vi "Mutate Multi FPGA.vi"(6 "Force (F)":bool, 8 "error in (no error)":errorcluster, 11 "Device Ref in":T1 format="%.0x") -> (0 "error out":errorcluster, 3 "Device Ref out":T1 format="%.0x")   [LabVIEW 2015, in "Engine Simulation Toolkit System Explorer.lvlib"]
uses:
  Engine Simulation Toolkit System Explorer.lvlib
  <vilib>/NI Veristand/Custom Device API/Custom Device Item Ref.ctl
  Shared/Channel.ctl
  <vilib>/NI Veristand/Custom Device API/Custom Device Channel Type.ctl
  Shared/Properties.vi
  Shared/Constants and GUIDs.vi
  <vilib>/NI Veristand/Custom Device API/Get Item Property (Boolean).vi
  <vilib>/NI Veristand/Custom Device API/Get Item Property (String).vi
  <vilib>/NI Veristand/Custom Device API/Set Item Property (String Array).vi
  <vilib>/NI Veristand/Custom Device API/Get Item Property (Dependent File).vi
  <vilib>/NI Veristand/Custom Device API/Set Item Property (String).vi
  <vilib>/NI Veristand/Custom Device Tools/Custom Device Utility Library/NI VeriStand - Search for All Items by GUID.vi
  <vilib>/NI Veristand/Custom Device API/Set Item Property (Boolean).vi
  Shared/Engine Simulation Toolkit Shared.lvlib
  <vilib>/NI VeriStand/Custom Device API/Custom Device API.lvlib
  <vilib>/NI VeriStand/Custom Device Tools/Custom Device Utility Library/Custom Device Utility Library.lvlib
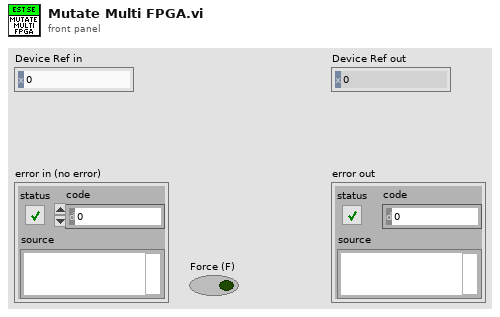
[diagram p1: front panel]
types:
  T1 = typedef "Custom Device API.lvlib/Custom Device Item Ref.ctl" = u64
  T2 = typedef "Engine Simulation Toolkit Shared.lvlib/Channel.ctl" = cluster{"Name":string, "Units":string, "Default":dbl, "Description":string, "Scalable":bool}
  T3 = typedef "Custom Device API.lvlib/Custom Device Channel Type.ctl" = enum16{"Input", "Output"}
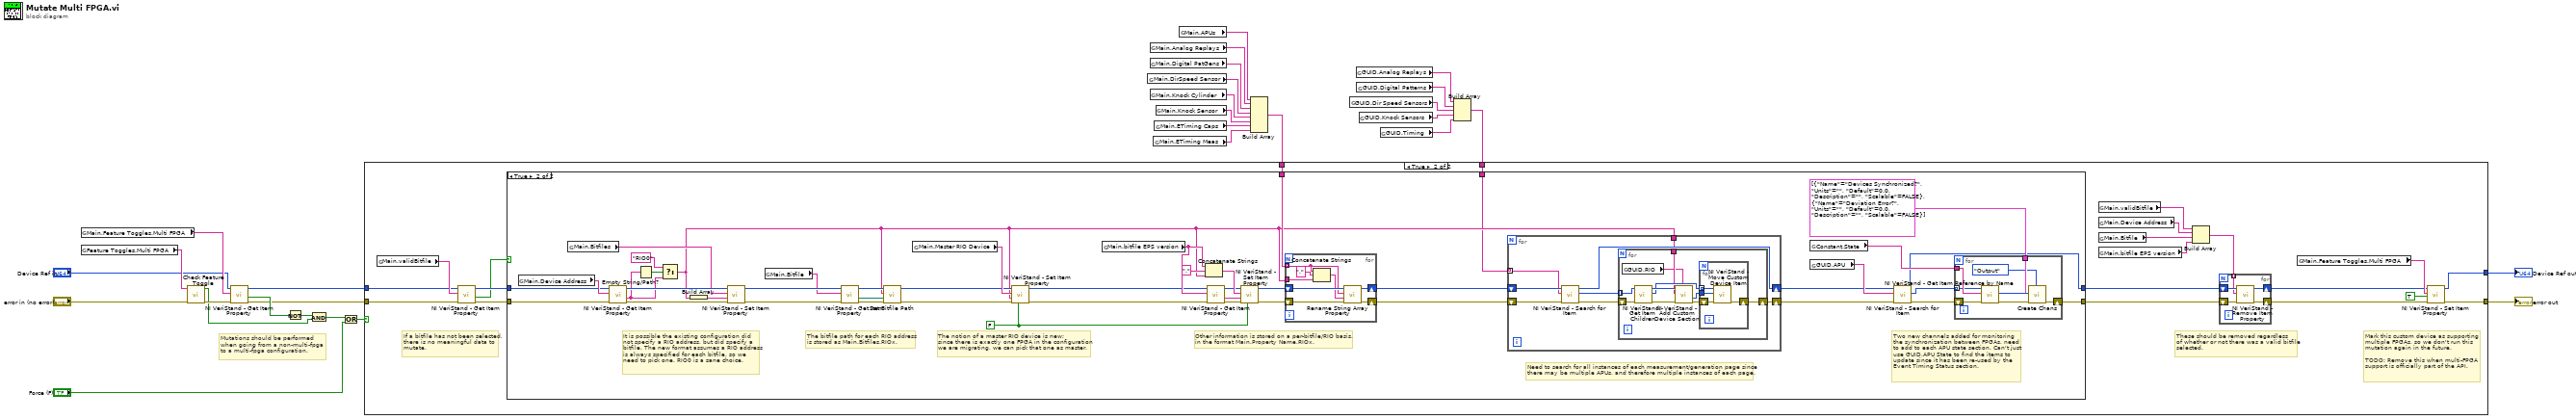
[diagram p0: block diagram]
diagram:
  # "Mutations should be performed\nwhen going from a non-multi-fpga\nto a multi-fpga configuration."
  n1 = global read "Properties.vi" "Main.Feature Toggles.Multi FPGA"() -> (w13:string)
  n2 = global read "Constants and GUIDs.vi" "Feature Toggles.Multi FPGA"() -> (w10:string)
  n3 = call "Check Feature Toggle.vi"("error in (no error)"="error in (no error)", "feature name"=w10) -> ("error out"=w9:errorcluster, "feature enabled"=w6:bool)  [unwired: 8 in]
  n4 = call-poly <vilib>:"NI VeriStand - Get Item Property.vi"("error in (no error)"=w9, "Property Name"=w13, "Item Ref in"="Device Ref in") -> ("error out"=w11:errorcluster, "Value"=w12:bool, "Item Ref out"=w1:T1)  [unwired: 5 in, 1 out]
  n5 = Not(x=w12) -> (.not. x?=w7:bool)
  n6 = And(x=w7, y=w6) -> (x .and. y?=w4:bool)
  n7 = Or(x=w4, y="Force (F)") -> (x .or. y?=w5:bool)
  n8 = global read "Properties.vi" "Main.DirSpeed Sensor"() -> (w26:string)
  n9 = global read "Properties.vi" "Main.Analog Replays"() -> (w24:string)
  n10 = global read "Properties.vi" "Main.Digital PatGens"() -> (w25:string)
  n11 = global read "Properties.vi" "Main.Knock Cylinder"() -> (w27:string)
  n12 = global read "Properties.vi" "Main.ETiming Meas"() -> (w29:string)
  n13 = global read "Properties.vi" "Main.ETiming Caps"() -> (w28:string)
  n14 = global read "Properties.vi" "Main.Knock Sensor"() -> (w30:string)
  n15 = global read "Properties.vi" "Main.APUs"() -> (w23:string)
  n16 = Build Array(w23, w24, w25, w26, w27, w30, w28, w29) -> (w22:string[])
  n17 = global read "Constants and GUIDs.vi" "GUID.Dir Speed Sensors"() -> (w19:string)
  n18 = global read "Constants and GUIDs.vi" "GUID.Analog Replays"() -> (w17:string)
  n19 = global read "Constants and GUIDs.vi" "GUID.Digital Patterns"() -> (w18:string)
  n20 = global read "Constants and GUIDs.vi" "GUID.Knock Sensors"() -> (w20:string)
  n21 = global read "Constants and GUIDs.vi" "GUID.Timing"() -> (w21:string)
  n22 = Build Array(w17, w18, w19, w20, w21) -> (w16:string[])
  n23 = case shown="True" w5 {
    tunnel: w22 -> [_ w53]
    tunnel: w11 -> [w32 w51]
    tunnel: w16 -> [_ w48]
    tunnel: [w32 w34] -> w14
    tunnel: [w31 w35] -> w15
    tunnel: w1 -> [w31 w33]
    frame False {
    }
    frame True {
      # "Mark this custom device as supporting\nmultiple FPGAs, so we don't run this\nmutation again in the future.\n\nTODO: Remove this when multi-FPGA\nsupport is officially part of the API."
      # "These should be removed regardless\nof whether or not there was a valid bitfile\nselected."
      # "If a bitfile has not been selected,\nthere is no meaningful data to\nmutate."
      n24 = global read "Properties.vi" "Main.validBitfile"() -> (w52:string)
      n25 = call-poly <vilib>:"NI VeriStand - Get Item Property.vi"("error in (no error)"=w51, "Property Name"=w52, "Item Ref in"=w33) -> ("error out"=w50:errorcluster, "Value"=w47:bool, "Item Ref out"=w49:T1)  [unwired: 5 in, 1 out]
      n26 = case shown="True" w47 {
        tunnel: w50 -> [w54 w57]
        tunnel: w49 -> [w55 w56]
        tunnel: [w55 w58] -> w45
        tunnel: [w54 w65] -> w46
        tunnel: w53 -> [_ w82]
        tunnel: w48 -> [_ w67]
        frame False {
        }
        frame True {
          w71 = FALSE ("Binary String (T)")
          # "Two new channels added for monitoring\nthe synchronization between FPGAs, need\nto add to each APU state section. Can't just\nuse GUID.APU State to find the items to\nupdate since it has been re-used by the \nEvent Timing Status section."
          # "Need to search for all instances of each measurement/generation page since\nthere may be multiple APUs, and therefore multiple instances of each page."
          # "Other information is stored on a per-bitfile/RIO basis,\nin the format Main.Property Name.RIOx."
          # "The notion of a master RIO device is new;\nsince there is exactly one FPGA in the configuration\nwe are migrating, we can pick that one as master."
          # "The bitfile path for each RIO address\nis stored as Main.Bitfiles.RIOx."
          # "It is possible the existing configuration did\nnot specify a RIO address, but did specify a\nbitfile. The new format assumes a RIO address\nis always specified for each bitfile, so we\nneed to pick one. RIO0 is a sane choice."
          n27 = global read "Properties.vi" "Main.Device Address"() -> (w91:string)
          n28 = global read "Properties.vi" "Main.Bitfiles"() -> (w83:string)
          n29 = call-poly <vilib>:"NI VeriStand - Get Item Property.vi"("error in (no error)"=w57, "Property Name"=w91, "Item Ref in"=w56) -> ("error out"=w97:errorcluster, "Value"=w80:string, "Item Ref out"=w98:T1)  [unwired: 5 in, 1 out]
          n30 = Empty String/Path?(string/path=w80) -> (empty?=w81:bool)
          n31 = Select(t="RIO0", s=w81, f=w80) -> (s? t:f=w70:string)
          n32 = Build Array(w70) -> (w99:string[])
          n33 = call-poly <vilib>:"NI VeriStand - Set Item Property.vi"("error in (no error)"=w97, "Value"=w99, "Property Name"=w83, "Item Ref in"=w98) -> ("error out"=w92:errorcluster, "Item Ref out"=w93:T1)  [unwired: 5 in, 1 out]
          n34 = global read "Properties.vi" "Main.Bitfile"() -> (w90:string)
          n35 = call-poly <vilib>:"NI VeriStand - Get Item Property.vi"("error in (no error)"=w92, "Property Name"=w90, "Item Ref in"=w93) -> ("error out"=w96:errorcluster, "Path"=w95:path, "Item Ref out"=w94:T1)  [unwired: 4 in, 2 out]
          n36 = call "Set Bitfile Path.vi"("error in (no error)"=w96, "Bitfile Path in"=w95, "RIO Device Address in"=w70, "Item Ref in"=w94) -> ("error out"=w74:errorcluster, "Item Ref out"=w73:T1)  [unwired: 6 in]
          n37 = global read "Properties.vi" "Main.Master RIO Device"() -> (w76:string)
          n38 = call-poly <vilib>:"NI VeriStand - Set Item Property.vi"("Binary String (T)"=w71, "error in (no error)"=w74, "Value"=w70, "Property Name"=w76, "Item Ref in"=w73) -> ("error out"=w75:errorcluster, "Item Ref out"=w72:T1)  [unwired: 4 in, 1 out]
          n39 = global read "Properties.vi" "Main.bitfile EPS version"() -> (w85:string)
          n40 = Concatenate Strings(w85, "." ("string"), w70) -> (w86:string)
          n41 = call-poly <vilib>:"NI VeriStand - Get Item Property.vi"("error in (no error)"=w75, "Property Name"=w85, "Item Ref in"=w72) -> ("error out"=w88:errorcluster, "Value"=w87:string, "Item Ref out"=w84:T1)  [unwired: 5 in, 1 out]
          n42 = call-poly <vilib>:"NI VeriStand - Set Item Property.vi"("Binary String (T)"=w71, "error in (no error)"=w88, "Value"=w87, "Property Name"=w86, "Item Ref in"=w84) -> ("error out"=w78:errorcluster, "Item Ref out"=w77:T1)  [unwired: 4 in, 1 out]
          n43 = for {
            tunnel: w70 -> [w136]
            tunnel: w82 -> [w133] mode=indexing
            shift-right: [w131] -> w68
            shift-left: w78 -> [w135]
            shift-right: [w130] -> w69
            shift-left: w77 -> [w134]
            n44 = Concatenate Strings(w133, "." ("string"), w136) -> (w132:string)
            n45 = call "Rename String Array Property.vi"("error in (no error)"=w135, "New Name"=w132, "Old Name"=w133, "Item Ref in"=w134) -> ("error out"=w131:errorcluster, "Item Ref out"=w130:T1)  [unwired: 6 in]
          }
          n46 = for {
            tunnel: w70 -> [w108]
            shift-right: [w111] -> w60
            shift-left: w68 -> [w112]
            shift-right: [w110] -> w61
            shift-left: w69 -> [w113]
            tunnel: w67 -> [w109] mode=indexing
            n47 = call-poly <vilib>:"NI VeriStand - Search for Item.vi"("error in"=w112, "Item GUID"=w109, "Section Ref in"=w113) -> ("error out"=w114:errorcluster, "Item Refs"=w115:T1[], "Section Ref out"=w110:T1)  [unwired: 5 in, 1 out]
            n48 = for {
              tunnel: w115 -> [w125] mode=indexing
              tunnel: w108 -> [w118]
              shift-right: [w116] -> w111
              shift-left: w114 -> [w122]
              n49 = global read "Constants and GUIDs.vi" "GUID.RIO"() -> (w117:string)
              n50 = call <vilib>:"NI VeriStand - Get Item Children.vi"("error in (no error)"=w122, "Item Ref in"=w125) -> ("error out"=w124:errorcluster, "Child Refs"=w119:T1[], "Item Ref out"=w123:T1)  [unwired: 6 in, 1 out]
              n51 = call <vilib>:"NI VeriStand - Add Custom Device Section.vi"("GUID (Default Section)"=w117, "error in (no error)"=w124, "Section Name"=w118, "Parent Ref in"=w123) -> ("error out"=w120:errorcluster, "Section Ptr"=w121:T1)  [unwired: 4 in, 2 out]
              n52 = for {
                tunnel: w121 -> [w129]
                tunnel: w119 -> [w127] mode=indexing
                shift-right: [w126] -> w116
                shift-left: w120 -> [w128]
                n53 = call <vilib>:"NI VeriStand - Move Custom Device Item.vi"("error in (no error)"=w128, "New Parent Ref in"=w129, "Item Ref in"=w127) -> ("error out"=w126:errorcluster)  [unwired: 6 in, 2 out]
              }
            }
          }
          n54 = global read "Constants and GUIDs.vi" "Constant.State"() -> (w66:string)
          n55 = global read "Constants and GUIDs.vi" "GUID.APU"() -> (w62:string)
          n56 = call-poly <vilib>:"NI VeriStand - Search for Item.vi"("error in"=w60, "Item GUID"=w62, "Section Ref in"=w61) -> ("error out"=w63:errorcluster, "Item Refs"=w59:T1[], "Section Ref out"=w58:T1)  [unwired: 5 in, 1 out]
          n57 = for {
            tunnel: w66 -> [w107]
            tunnel: T2[] [{"Name"="Devices Synchronized?", "Units"="", "Default"=0.0, "Description"="", "Scalable"=FALSE}, {"Name"="Deviation Error?", "Units"="", "Default"=0.0, "Description"="", "Scalable"=FALSE}] ("ChanList.APU State") -> [w103]
            tunnel: w59 -> [w100] mode=indexing
            shift-right: [w105] -> w65
            shift-left: w63 -> [w101]
            n58 = call <vilib>:"NI VeriStand - Get Item Reference by Name.vi"("error in (no error)"=w101, "Item Name"=w107, "Parent Ref in"=w100) -> ("error out"=w106:errorcluster, "Item Ref"=w104:T1)  [unwired: 5 in, 2 out]
            n59 = call "Create Chans.vi"("Type"=Custom_Device_Channel_Type."Output", "error in (no error)"=w106, "Channels"=w103, "Section Ptr"=w104) -> ("error out"=w105:errorcluster)  [unwired: 4 in, 3 out]
          }
        }
      }
      n60 = global read "Properties.vi" "Main.validBitfile"() -> (w43:string)
      n61 = global read "Properties.vi" "Main.Device Address"() -> (w44:string)
      n62 = global read "Properties.vi" "Main.Bitfile"() -> (w42:string)
      n63 = global read "Properties.vi" "Main.bitfile EPS version"() -> (w41:string)
      n64 = Build Array(w43, w44, w42, w41) -> (w40:string[])
      n65 = for {
        shift-right: [w139] -> w38
        shift-left: w45 -> [w141]
        tunnel: w40 -> [w138] mode=indexing
        shift-right: [w140] -> w37
        shift-left: w46 -> [w142]
        n66 = call <vilib>:"NI VeriStand - Remove Item Property.vi"("error in (no error)"=w142, "Property Name"=w138, "Item Ref in"=w141) -> ("error out"=w140:errorcluster, "Item Ref out"=w139:T1)  [unwired: 6 in, 1 out]
      }
      n67 = global read "Properties.vi" "Main.Feature Toggles.Multi FPGA"() -> (w39:string)
      n68 = call-poly <vilib>:"NI VeriStand - Set Item Property.vi"("error in (no error)"=w37, "Value"=TRUE, "Property Name"=w39, "Item Ref in"=w38) -> ("error out"=w34:errorcluster, "Item Ref out"=w35:T1)  [unwired: 5 in, 1 out]
    }
  }
  "Device Ref out" <- w15
  "error out" <- w14
